vi "Barcode Scanner1.vi"() -> ()   [LabVIEW 2015]
uses:
  <vilib>/Instr/_visa.llb/VISA Configure Serial Port (Instr).vi
panel:
  out "exit":bool
  out "error out 2":errorcluster
  out "read buffer":string
  in  "stop":bool
  out "error out":errorcluster
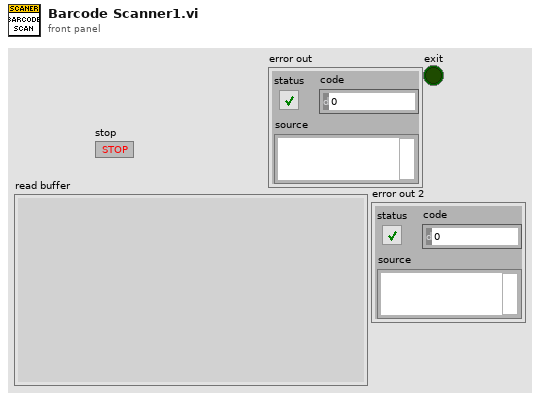
[diagram p1: front panel]
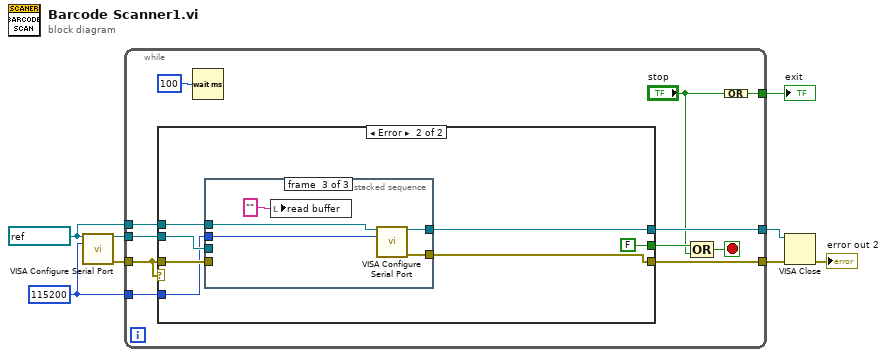
[diagram p0: block diagram]
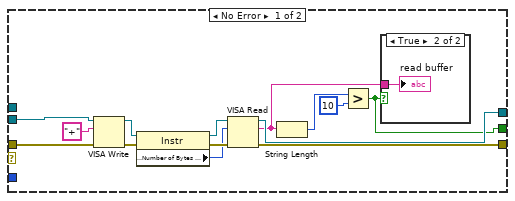
[diagram p2: hidden frame]
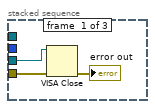
[diagram p4: hidden frame]
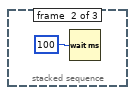
[diagram p5: hidden frame]
diagram:
  w3 = u32 115200 ("baud rate (9600)")
  w4 = refnum<visa-resource-name> "COM2" ("VISA resource name")
  n1 = call-poly "VISA Configure Serial Port"("VISA resource name"=w4, "baud rate (9600)"=w3) -> ("VISA resource name out"=w8:refnum<visa-resource-name>, "error out"=w7:errorcluster)  [unwired: 12 in]
  n2 = while {
    tunnel: w8 -> [w19]
    tunnel: w7 -> [w16]
    tunnel: [w18] -> w6
    tunnel: [w17] -> w5
    tunnel: w4 -> [w15]
    tunnel: w3 -> [w14]
    tunnel: [w9] -> w1
    stop <- w12 stop-if-true
    n3 = case shown="Error" w16 {
      tunnel: w19 -> [w33 w41]
      tunnel: w16 -> [w32 w40]
      tunnel: [w31 w37] -> w18
      tunnel: [w30 w36] -> w17
      tunnel: w15 -> [_ w39]
      tunnel: w14 -> [_ w38]
      tunnel: [w20 FALSE] -> w11
      frame No Error {
        n4 = VISA Write(VISA resource name=w33, write buffer="+", error in (no error)=w32) -> (VISA resource name out=w28:refnum<visa-resource-name>, error out=w29:errorcluster)  [unwired: 1 out]
        n5 = property class="Instr"(reference=w28, error in=w29) -> (reference out=w27:refnum<visa-resource-name>, error out=w26:errorcluster, "Serial Settings:Number of Bytes at Serial Port"=w25:u32)
        n6 = VISA Read(VISA resource name=w27, byte count=w25, error in (no error)=w26) -> (VISA resource name out=w31:refnum<visa-resource-name>, read buffer=w21:string, error out=w30:errorcluster)  [unwired: 1 out]
        n7 = String Length(string=w21) -> (length=w23:i32)
        n8 = Greater?(x=w23, y=10) -> (0:w20:bool)
        n9 = case shown="True" w20 {
          tunnel: w21 -> [_ w34]
          frame False {
          }
          frame True {
            "read buffer" <- w34
          }
        }
      }
      frame Error {
        n10 = stacked-sequence {
          tunnel: w41 -> [w43 _ _]
          tunnel: w40 -> [w42 _ _]
          tunnel: w39 -> [_ _ w50]
          tunnel: w38 -> [_ _ w49]
          tunnel: [_ _ w48] -> w37
          tunnel: [_ _ w47] -> w36
          frame #0 {
            n11 = VISA Close(VISA resource name=w43, error in (no error)=w42) -> (error out=→"error out":errorcluster)
          }
          frame #1 {
            n12 = Wait (ms)(milliseconds to wait=u32 100) -> ()  [unwired: 1 out]
          }
          frame #2 {
            n13 = local write "read buffer"("" ("read buffer")) -> ()
            n14 = call-poly "VISA Configure Serial Port"("VISA resource name"=w50, "baud rate (9600)"=w49) -> ("VISA resource name out"=w48:refnum<visa-resource-name>, "error out"=w47:errorcluster)  [unwired: 12 in]
          }
        }
      }
    }
    n15 = Wait (ms)(milliseconds to wait=u32 100) -> ()  [unwired: 1 out]
    n16 = Compound Arithmetic op=OR(w11, "stop") -> (w12:bool)
    n17 = Compound Arithmetic op=OR("stop") -> (w9:bool)
  }
  "exit" <- w1
  n18 = VISA Close(VISA resource name=w6, error in (no error)=w5) -> (error out=→"error out 2":errorcluster)
